vi "Create Config Hash.vi"(8 "error in (no error)":errorcluster, 11 "VolatusConfig in":refnum<class "VolatusConfig.lvclass">) -> (0 "error out":errorcluster, 3 "VolatusConfig out":refnum<class "VolatusConfig.lvclass">)   [LabVIEW 2023, in "VolatusConfig.lvlib" / "VolatusConfig.lvclass"]
uses:
  VolatusConfig.lvclass
  Meta Name.ctl
  VolatusConfig.lvclass/VolatusConfig.ctl
  lv-cdm/CDM-Config/Config Element/Config Element.lvclass
  VolatusConfig.lvlib
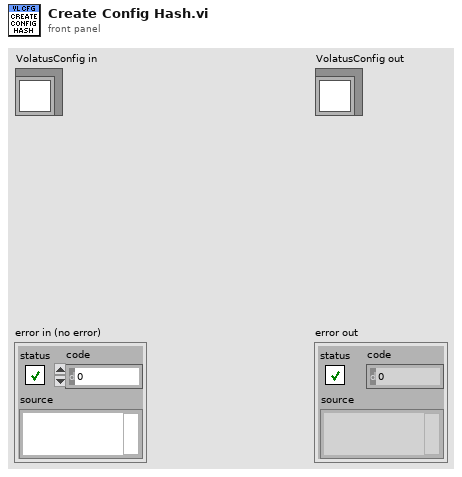
[diagram p1: front panel]
types:
  T1 = typedef "VolatusConfig.lvlib/Meta Name.ctl" = enum16{"VL_Type", "VL_Node_IP", "VL_Node_Type", "VL_Task_Type", "VL_Group_Type", "VL_Channel_Type", "VL_Channel_DataType", "VL_Config_Version", "VL_Overlay_Type", "VL_Config_Hash"}
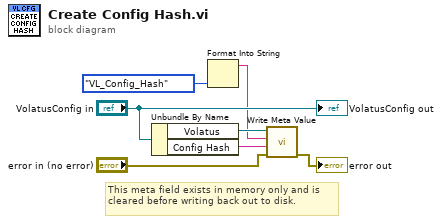
[diagram p0: block diagram]
diagram:
  # "This meta field exists in memory only and is cleared before writing back out to disk."
  n1 = Unbundle By Name("VolatusConfig in") -> ("Volatus"=w6:refnum<class "Config Element.lvclass">, "Config Hash"=w5:string)
  n2 = Format Into String(Meta_Name."VL_Config_Hash" ("Meta Name")) -> (resulting string=w3:string)  [unwired: 3 in, 1 out]
  n3 = call "Write Meta Value.vi"("error in (no error)"="error in (no error)", "Meta Value"=w5, "Meta Name"=w3, "Config Element in"=w6) -> ("error out"=→"error out":errorcluster)  [unwired: 6 in, 1 out]
  "VolatusConfig out" <- "VolatusConfig in"
